vi "Build.vi"(8 "error in (no error)":errorcluster, 11 "Build in":refnum<class "AB_Application.lvclass">) -> (0 "error out":errorcluster, 1 "GeneratedFiles":path[](array[path]), 2 "GeneratedDirectories":path[](array[path]), 3 "Build out":refnum<class "AB_Application.lvclass">, 4 "GeneratedFileGUIDs":string[](array[string]), 5 "OutputDirectory":path, 7 "Dependencies":T1[](array[typedef]))   [LabVIEW 2020, in "AB_Application.lvclass"]
uses:
  <vilib>/AppBuilder/AB_Classes/Application/AB_Application.lvclass
  e:/builds/penguin/labview/branches/2020/dev/dist/vi.lib/AppBuilder/AB_Classes/Build/AB_Build.lvclass
  <vilib>/AppBuilder/AB_Dependency.ctl
  <vilib>/Utility/lvfile.llb/LVFileType.ctl
  <vilib>/AppBuilder/AB_Classes/TargetFile/AB_Targetfile.lvclass
  <vilib>/AppBuilder/AB_Classes/Build/AB_Build.lvclass
  <vilib>/Utility/lvfile.llb/NI_FileType.lvlib
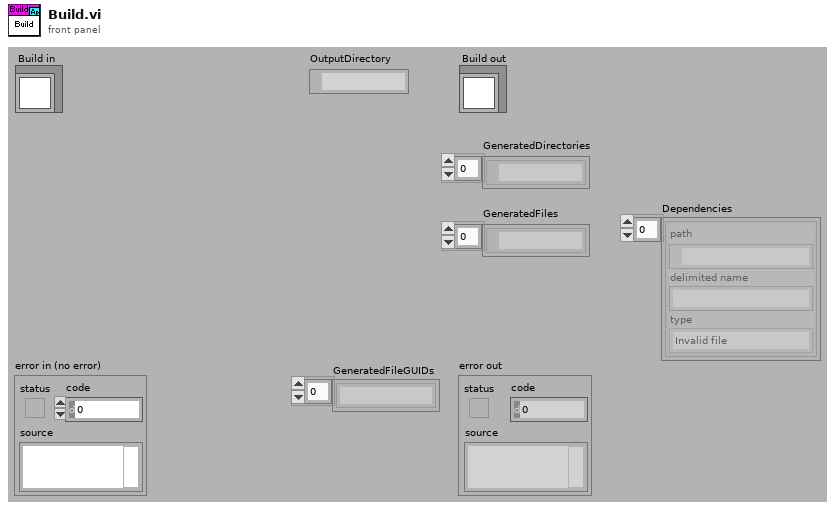
[diagram p1: front panel]
types:
  T1 = typedef "AB_Dependency.ctl" = cluster{"path":path, "delimited name":string, "type":T2}
  T2 = typedef "NI_FileType.lvlib/LVFileType.ctl" = enum32{"Invalid file", "Unknown type", "Instrument", "Control", "Polymorphic VI", "Project", "Library", "LVClass", "XControl", "XNode", "Shared library", ".NET assembly", "ActiveX interface", "CIN", "Run-time menu", "Palette menu", "Help file", "LLB", "XNode Edit Dependency", "Class Private Data Control", "Statechart", "MathScript .m file", "Ladder Diagram", "LVLibp", "XNode Build Dependency"}
  T3 = enum32{"invalid OS target", "Mac OS", "Windows 3.1", "Windows 95/NT", "Solaris 1", "Solaris 2", "HP-UX", "PowerMAX", "Linux", "Irix", "Rhapsody", "BeOS", "AIX", "OSF1", "VxWorks", "PharLap", "Carbon", "RTX", "Windows x64", "Linux x64", "Mac OS X x64"}
  T4 = typedef "AB_Build.ctl" = cluster{"buildSpecName":string, "buildSpecDescription":string, "destinations":refnum<class "AB_Destination.lvclass">[], "exclusionOption":T5, "defaultLanguage":string, "supportedLanguages":string[], "excludedDirectories":path[], "buildContext":refnum<vi>, "buildObject":T6, "preview":bool, "programatic":bool, "progressBarEvents":T7, "userLog_Path":path, "preActionID":string, "preAction_Path":path, "postActionID":string, "postAction_Path":path, "eng_checkForBrokenVIs?":bool, "eng_verboseLinkerErrors?":bool, "localDest_Path":path, "targetDest_Path":path, "removeVIObject":u16, "cache":refnum<class "PreviewCache.lvclass">, "use cache":bool, "previewCache_ID":string, "buildCache_ID":string, "eng_TempLocalDest_Path":path, "eng_collectDependencies?":bool, "versionInfo":cluster{"buildVersion":cluster{"major":u16, "minor":u16, "patch":u16, "build":u16}, "autoIncrement":bool}, "eng_enableVIChecksums":bool}
  T5 = typedef "AB_Exclusion_Option.ctl" = cluster{"typedefs":bool, "polymorphicVIs":bool, "unusedLibraryItems":bool, "modifyLibraryFile":bool, "edit-timeDependencies":bool, "inlineVIs":bool, "dependent PPLs":bool, "dependent DLLs":bool}
  T6 = typedef "ItemRef.ctl" = u64
  T7 = typedef "provcom_ProgressBar_Events.ctl" = cluster{"newJob":refnum<user-event>, "newItem":refnum<user-event>, "errorMsg":T8, "cancel":refnum<user-event>}
  T8 = typedef "mxLvBuildError.ctl" = refnum<user-event>
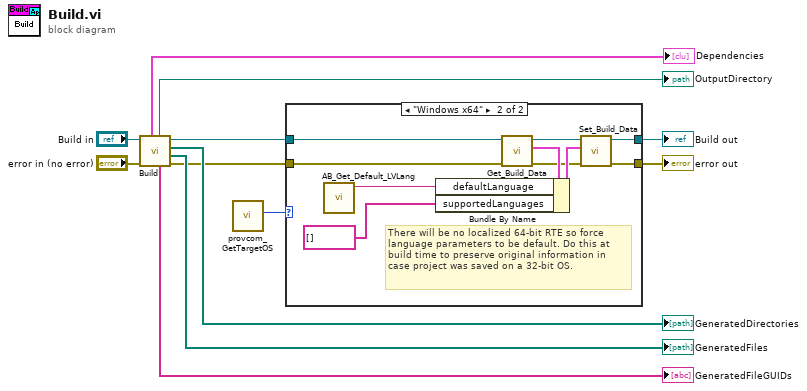
[diagram p0: block diagram]
diagram:
  n1 = call-parent "Build.vi"("error in (no error)"="error in (no error)", "Build in"="Build in") -> ("error out"=w4:errorcluster, "GeneratedFiles"=→"GeneratedFiles":path[], "GeneratedDirectories"=→"GeneratedDirectories":path[], "Build out"=w5:refnum<class "AB_Application.lvclass">, "GeneratedFileGUIDs"=→"GeneratedFileGUIDs":string[], "OutputDirectory"=→"OutputDirectory":path, "Dependencies"=→"Dependencies":T1[])  [unwired: 3 out]
  n2 = call <resource>:"provcom_GetTargetOS.vi"() -> ("App.TargetOS"=w6:T3)  [unwired: 11 out]
  n3 = case shown="\"Windows x64\"" w6 {
    tunnel: w5 -> [w14 w24]
    tunnel: w4 -> [w13 w20]
    tunnel: [w14 w22] -> w3
    tunnel: [w13 w21] -> w2
    frame Default {
    }
    frame "Windows x64" {
      # "There will be no localized 64-bit RTE so force language parameters to be default. Do this at build time to preserve original information in case project was saved on a 32-bit OS."
      n4 = call <vilib>:"AB_Get_Default_LVLang.vi"() -> ("env_language"=w16:string)  [unwired: 1 in, 10 out]
      n5 = call <vilib>:"Get_Build_Data.vi"("error in (no error)"=w20, "Class in"=w24) -> ("error out"=w17:errorcluster, "data"=w19:T4, "Class out"=w23:refnum<class "AB_Application.lvclass">)  [unwired: 7 out]
      n6 = Bundle By Name(cluster=w19, "defaultLanguage"=w16, "supportedLanguages"=string[] []) -> (w18:T4)
      n7 = call <vilib>:"Set_Build_Data.vi"("error in (no error)"=w17, "data"=w18, "Class in"=w23) -> ("error out"=w21:errorcluster, "Class out"=w22:refnum<class "AB_Application.lvclass">)  [unwired: 7 out]
    }
  }
  "error out" <- w2
  "Build out" <- w3
